vi "自动打签.vi"() -> ()   [LabVIEW 2018]
uses:
  <userlib>/snap7/Snap7.lvlib
panel:
  in  "选择班次":string(combo)
  in  "型号选择":string(combo)
  in  "停止":bool
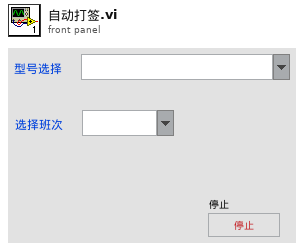
[diagram p1: front panel]
types:
  T1 = enum16{"读取布尔", "写入布尔", "读取无符号整形", "写入无符号整形", "读取有符号整形", "写入有符号整形", "读取单精度", "写入单精度", "读取双精度", "写入双精度", "读取字符串", "写入字符串", "读取字符数组", "写入字符数组"}
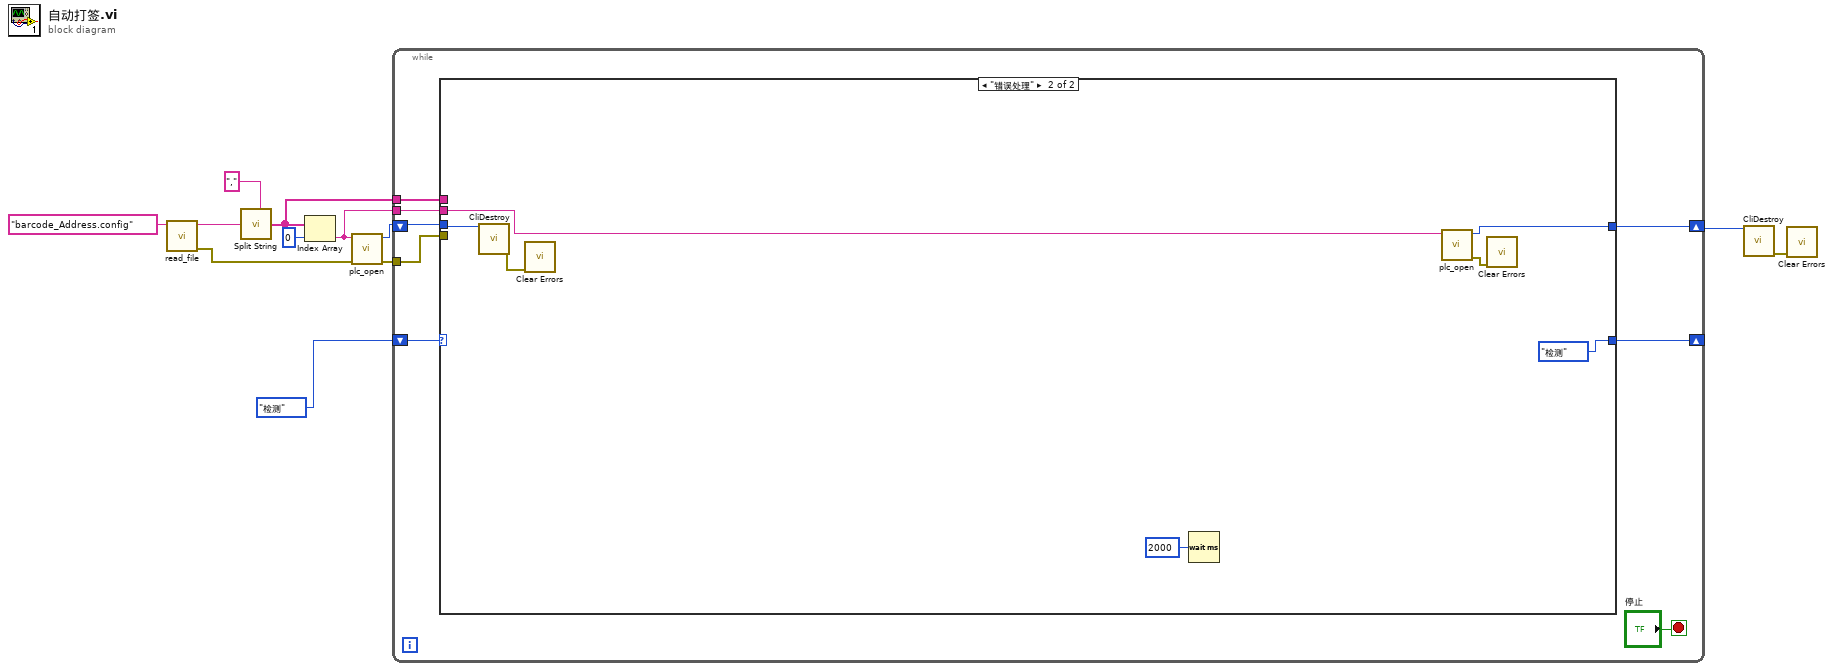
[diagram p0: block diagram]
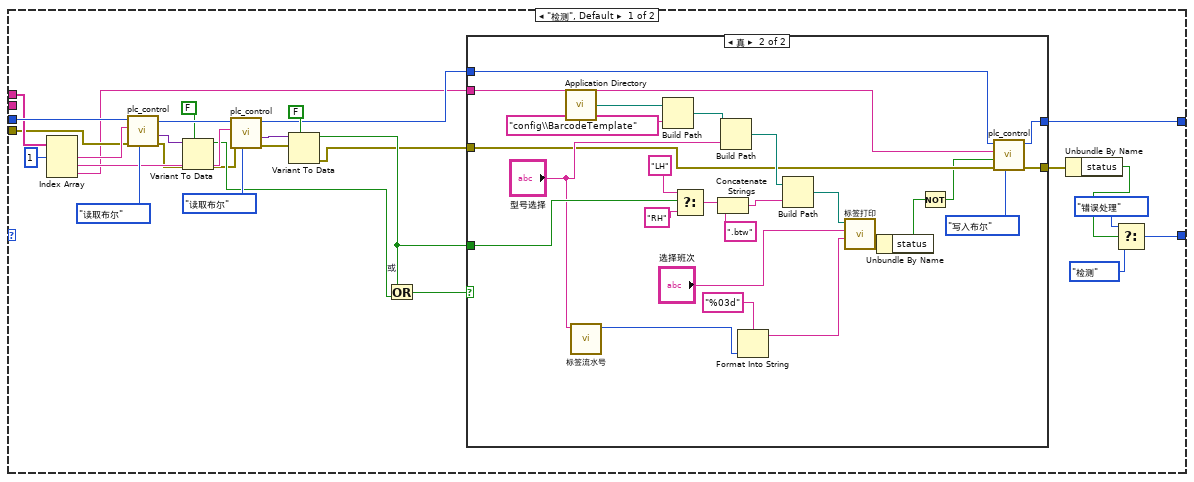
[diagram p2: hidden frame]
diagram:
  n1 = call "read_file.vi"("文件名"="barcode_Address.config") -> ("错误输出"=w6:errorcluster, "输出"=w12:string)  [unwired: 9 in]
  n2 = call <vilib>:"Split String.vi"("Split Pattern"=",", "Input String"=w12) -> ("Split String"=w8:string[])  [unwired: 5 in]
  n3 = Index Array(array=w8, index=0 ("索引")) -> (element=w2:string)
  n4 = call "plc_open.vi"("error in (no error)"=w6, "Address"=w2) -> ("error out"=w7:errorcluster, "ref out"=w9:u64)  [unwired: 8 in]
  n5 = while {
    tunnel: w8 -> [w18]
    tunnel: w7 -> [w17]
    shift-right: [w16] -> w4
    shift-left: w9 -> [w19]
    tunnel: w2 -> [w14]
    shift-right: [w13] -> _
    shift-left: enum16{"检测", "错误处理"}."检测" -> [w15]
    stop <- "停止" stop-if-true
    n6 = case shown="\"错误处理\"" w15 {
      tunnel: w19 -> [w48 w82]
      tunnel: w18 -> [w47 _]
      tunnel: w17 -> [w41 _]
      tunnel: [w31 w80] -> w16
      tunnel: w14 -> [_ w81]
      tunnel: [w26 enum16{"检测", "错误处理"}."检测"] -> w13
      frame "检测", Default {
        n7 = Index Array(array=w47, index #1=1 ("索引")) -> (element #1=w45:string, element #2=w42:string, element #3=w30:string)  [unwired: 2 in]
        n8 = call "plc_control.vi"("枚举"=T1."读取布尔", "error in (no error)"=w41, "地址"=w45, "ref in"=w48) -> ("error out"=w24:errorcluster, "Variant"=w39:variant, "ref out"=w40:u64)  [unwired: 5 in]
        n9 = Variant To Data(error in=w24, type=FALSE, Variant=w39) -> (data=w35:bool, error out=w23:errorcluster)
        n10 = call "plc_control.vi"("枚举"=T1."读取布尔", "error in (no error)"=w23, "地址"=w42, "ref in"=w40) -> ("error out"=w22:errorcluster, "Variant"=w36:variant, "ref out"=w32:u64)  [unwired: 5 in]
        n11 = Variant To Data(error in=w22, type=FALSE, Variant=w36) -> (data=w33:bool, error out=w21:errorcluster)
        n12 = Or "或"(x=w33, y=w35) -> (x .or. y?=w34:bool)
        n13 = case shown="真" w34 {
          tunnel: w33 -> [_ w68]
          tunnel: w32 -> [w50 w58]
          tunnel: [w50 w57] -> w31
          tunnel: w21 -> [w49 w56]
          tunnel: [w49 w55] -> w29
          tunnel: w30 -> [_ w51]
          frame False {
          }
          frame True {
            n14 = call <vilib>:"Application Directory.vi"() -> ("Application Directory"=w75:path)
            n15 = call "标签流水号.vi"("选择的型号"="型号选择") -> ("数值"=w61:i32)  [unwired: 10 in]
            n16 = Build Path(base path=w75, name or relative path="config\\BarcodeTemplate" ("名称或相对路径")) -> (appended path=w73:path)
            n17 = Select(t="LH" ("名称（未命名）"), s=w68, f="RH" ("名称（未命名）")) -> (s? t:f=w70:string)
            n18 = Concatenate Strings(w70, ".btw" ("字符串")) -> (w66:string)
            n19 = Build Path(base path=w73, name or relative path="型号选择") -> (appended path=w67:path)
            n20 = Format Into String(format string="%03d" ("格式字符串"), w61) -> (resulting string=w60:string)  [unwired: 2 in, 1 out]
            n21 = Build Path(base path=w67, name or relative path=w66) -> (appended path=w65:path)
            n22 = call "标签打印.vi"("流水号（3位）"=w60, "班次"="选择班次", "路径"=w65) -> ("error out"=w54:errorcluster)  [unwired: 7 in, 1 out]
            n23 = Unbundle By Name(w54) -> ("status"=w53:bool)
            n24 = Not(x=w53) -> (.not. x?=w52:bool)
            n25 = call "plc_control.vi"("枚举"=T1."写入布尔", "error in (no error)"=w56, "变体"=w52, "地址"=w51, "ref in"=w58) -> ("error out"=w55:errorcluster, "ref out"=w57:u64)  [unwired: 4 in, 1 out]
          }
        }
        n26 = Unbundle By Name(w29) -> ("status"=w28:bool)
        n27 = Select(t=enum16{"检测", "错误处理"}."错误处理", s=w28, f=enum16{"检测", "错误处理"}."检测") -> (s? t:f=w26:enum16{"检测", "错误处理"})
      }
      frame "错误处理" {
        n28 = call <userlib>:"CliDestroy.vi"("ref in"=w82) -> ("error out"=w78:errorcluster)  [unwired: 14 in]
        n29 = call <vilib>:"Clear Errors.vi"("error in (no error)"=w78) -> ()  [unwired: 5 in, 2 out]
        n30 = Wait (ms)(milliseconds to wait=u32 2000 ("等待时间（毫秒）")) -> ()  [unwired: 1 out]
        n31 = call "plc_open.vi"("Address"=w81) -> ("error out"=w79:errorcluster, "ref out"=w80:u64)  [unwired: 9 in]
        n32 = call <vilib>:"Clear Errors.vi"("error in (no error)"=w79) -> ()  [unwired: 5 in, 2 out]
      }
    }
  }
  n33 = call <userlib>:"CliDestroy.vi"("ref in"=w4) -> ("error out"=w1:errorcluster)  [unwired: 14 in]
  n34 = call <vilib>:"Clear Errors.vi"("error in (no error)"=w1) -> ()  [unwired: 5 in, 2 out]
